vi "Read Near Field Communication Trigger Time.vi"(8 "error in (no error)":errorcluster, 11 "VISA resource name":refnum<visa-resource-name>) -> (0 "error out":errorcluster, 1 "Timeout State":bool, 2 "Arm And Trigger Time (S)":dbl, 3 "VISA resource name out":refnum<visa-resource-name>)   [LabVIEW 2015, in "Agilent 2000 3000 X-Series.lvlib"]
doc: "Returns the timeout state and the time between the arm and the trigger.\n\n<b>Note:</b>\nThis VI is only applicable for 3000T, 4000 X-Series."
uses:
  Agilent 2000 3000 X-Series.lvlib
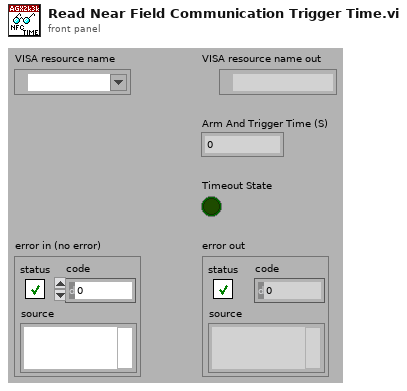
[diagram p1: front panel]
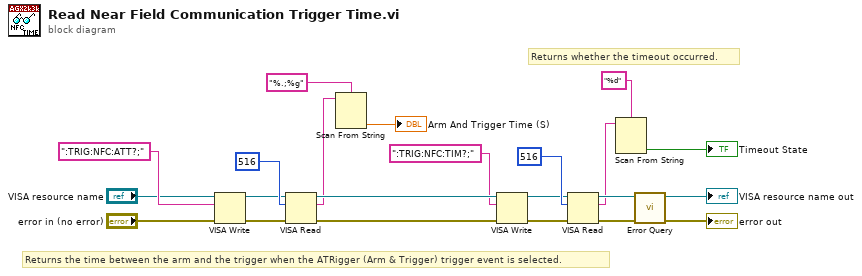
[diagram p0: block diagram]
diagram:
  # "Returns whether the timeout occurred."
  # "Returns the time between the arm and the trigger when the ATRigger (Arm & Trigger) trigger event is selected."
  n1 = VISA Write(VISA resource name="VISA resource name", write buffer=":TRIG:NFC:ATT?;", error in (no error)="error in (no error)") -> (VISA resource name out=w18:refnum<visa-resource-name>, error out=w17:errorcluster)  [unwired: 1 out]
  n2 = VISA Read(VISA resource name=w18, byte count=516, error in (no error)=w17) -> (VISA resource name out=w13:refnum<visa-resource-name>, read buffer=w5:string, error out=w12:errorcluster)  [unwired: 1 out]
  n3 = Scan From String(format string="%.;%g", input string=w5) -> (output 1=→"Arm And Trigger Time (S)":dbl)  [unwired: 3 in, 3 out]
  n4 = VISA Write(VISA resource name=w13, write buffer=":TRIG:NFC:TIM?;", error in (no error)=w12) -> (VISA resource name out=w15:refnum<visa-resource-name>, error out=w14:errorcluster)  [unwired: 1 out]
  n5 = VISA Read(VISA resource name=w15, byte count=516, error in (no error)=w14) -> (VISA resource name out=w10:refnum<visa-resource-name>, read buffer=w3:string, error out=w9:errorcluster)  [unwired: 1 out]
  n6 = Scan From String(format string="%d", input string=w3) -> (output 1=→"Timeout State":bool)  [unwired: 3 in, 3 out]
  n7 = call "Error Query.vi"("error in (no error)"=w9, "VISA resource name"=w10) -> ("error out"=→"error out":errorcluster, "VISA resource name out"=→"VISA resource name out":refnum<visa-resource-name>)  [unwired: 6 in, 2 out]
